vi "Check File Path.vi"(9 "Auto-Increment File Name":bool=TRUE, 11 "Camera Settings In":T1={"Exposure Time (ms)"=100.0, "Binning"=enum."2x2", "Scan Mode"=0, "Frames to Acquire"=1000.0, "Pixel Correction"=FALSE, "Frames to Skip"=0, "File Path"=path "", "Duty cycle"=0.0, "ALEX"=FALSE, "Shutter Enable"=[], "fluidics trigger frame"=0, "Bit Depth"=16, "Image Width (px)"=0, "Image Height (px)"=0, "Horizontal Offset (px)"=0, "Vertical Offset (px)"=0} {"fluidics trigger frame" max=60000 step=1; "Exposure Time (ms)" min=1.0 max=10000.0 step=1.0}) -> (1 "Ok":bool, 3 "Camera Settings Out":T1={"Exposure Time (ms)"=100.0, "Binning"=enum."2x2", "Scan Mode"=0, "Frames to Acquire"=1000.0, "Pixel Correction"=FALSE, "Frames to Skip"=0, "File Path"=path "", "Duty cycle"=0.0, "ALEX"=FALSE, "Shutter Enable"=[], "fluidics trigger frame"=0, "Bit Depth"=16, "Image Width (px)"=0, "Image Height (px)"=0, "Horizontal Offset (px)"=0, "Vertical Offset (px)"=0} {"fluidics trigger frame" max=60000 step=1; "Exposure Time (ms)" min=1.0 max=10000.0 step=1.0})   [LabVIEW 2023]
uses:
  Type Defs/Camera Settings.ctl
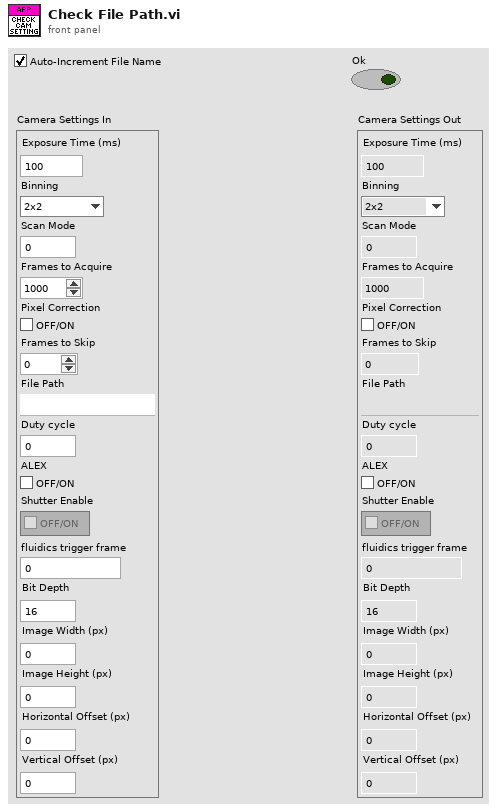
[diagram p1: front panel]
types:
  T1 = typedef "Camera Settings.ctl" = cluster{"Exposure Time (ms)":dbl, "Binning":enum16{"1x1", "2x2", "4x4"}, "Scan Mode":i32, "Frames to Acquire":dbl, "Pixel Correction":bool, "Frames to Skip":u32, "File Path":path, "Duty cycle":dbl, "ALEX":bool, "Shutter Enable":bool[], "fluidics trigger frame":u16, "Bit Depth":u16, "Image Width (px)":u16, "Image Height (px)":u16, "Horizontal Offset (px)":u16, "Vertical Offset (px)":u16}
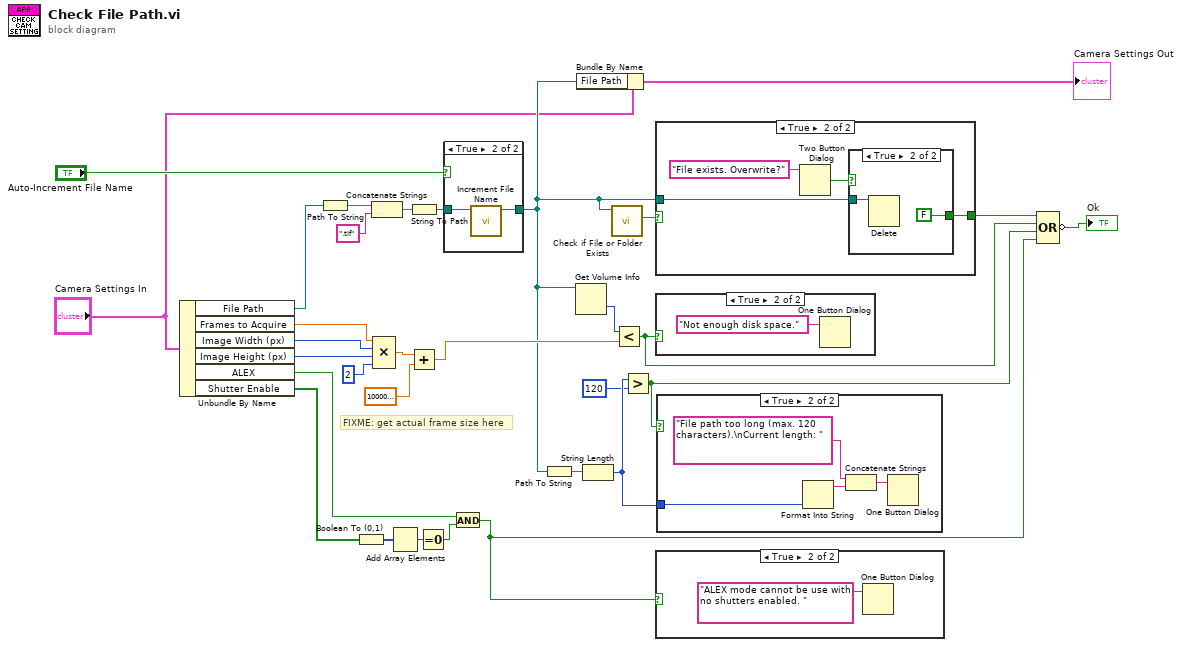
[diagram p0: block diagram]
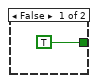
[diagram p5: hidden frame]
diagram:
  # "FIXME: get actual frame size here"
  n1 = Unbundle By Name("Camera Settings In") -> ("File Path"=w19:path, "Frames to Acquire"=w22:dbl, "Image Width (px)"=w10:u16, "Image Height (px)"=w9:u16, "ALEX"=w4:bool, "Shutter Enable"=w5:bool[])
  n2 = Path To String(path=w19) -> (string=w20:string)
  n3 = Boolean To (0,1)(Boolean=w5) -> (0, 1=w6:i16[])
  n4 = Concatenate Strings(w20, ".tif" ("string")) -> (w17:string)
  n5 = Compound Arithmetic op=MULTIPLY(w22, w10, w9, u16 2 ("value")) -> (w13:dbl)
  n6 = Add Array Elements(numeric array=w6) -> (sum=w3:i16)
  n7 = String To Path(string=w17) -> (path=w18:path)
  n8 = Add(x=w13, y=100000000.0 ("x")) -> (x+y=w28:dbl)
  n9 = Equal To 0?(x=w3) -> (x = 0?=w2:bool)
  n10 = case shown="True" "Auto-Increment File Name" {
    tunnel: w18 -> [w32 w34]
    tunnel: [w32 w33] -> w16
    frame False {
    }
    frame True {
      n11 = call "Increment File Name.vi"("Input Path"=w34) -> ("Output Path"=w33:path)  [unwired: 10 in]
    }
  }
  n12 = And(x=w4, y=w2) -> (x .and. y?=w1:bool)
  n13 = Path To String(path=w16) -> (string=w25:string)
  n14 = Get Volume Info(11:w16) -> (1:w24:i64)  [unwired: 1 in, 5 out]
  n15 = Bundle By Name(cluster="Camera Settings In", "File Path"=w16) -> (→"Camera Settings Out":T1)
  n16 = String Length(string=w25) -> (length=w27:i32)
  n17 = call <vilib>:"Check if File or Folder Exists.vi"("path"=w16) -> ("file or folder exists?"=w15:bool)  [unwired: 8 in, 2 out]
  n18 = Less?(x=w24, y=w28) -> (x < y?=w7:bool)
  n19 = Greater?(x=w27, y=120) -> (0:w11:bool)
  n20 = case shown="True" w15 {
    selector: w15 -> [w35 _]
    tunnel: [w35 w36] -> w29
    tunnel: w16 -> [_ w37]
    frame False {
    }
    frame True {
      n21 = Two Button Dialog(message="File exists. Overwrite?") -> (T button?=w38:bool)  [unwired: 2 in]
      n22 = case shown="True" w38 {
        tunnel: w37 -> [_ w42]
        tunnel: [TRUE FALSE] -> w36
        frame False {
        }
        frame True {
          n23 = Delete(path (use dialog)=w42) -> ()  [unwired: 4 in, 3 out]
        }
      }
    }
  }
  n24 = case shown="True" w7 {
    frame False {
    }
    frame True {
      n25 = One Button Dialog(message="Not enough disk space.") -> ()  [unwired: 1 in, 1 out]
    }
  }
  n26 = case shown="True" w1 {
    frame False {
    }
    frame True {
      n27 = One Button Dialog(message="ALEX mode cannot be use with no shutters enabled. ") -> ()  [unwired: 1 in, 1 out]
    }
  }
  n28 = case shown="True" w11 {
    tunnel: w27 -> [_ w45]
    frame False {
    }
    frame True {
      n29 = Format Into String(w45) -> (resulting string=w46:string)  [unwired: 3 in, 1 out]
      n30 = Concatenate Strings("File path too long (max. 120 characters).\nCurrent length: " ("message"), w46) -> (w47:string)
      n31 = One Button Dialog(message=w47) -> ()  [unwired: 1 in, 1 out]
    }
  }
  n32 = Compound Arithmetic op=OR(w29, w7, w11, w1) -> (invert →"Ok":bool)
